vi "xijk_select_best_filter_remove_NaN.vi"(8 "error in":errorcluster, 10 "table_input_1D":string[](array[string]), 11 "table_input_2D":string[][](array[string])) -> (0 "error out":errorcluster, 2 "table_output_1D":string[](array[string]), 3 "table_output_2D":string[][](array[string]))   [LabVIEW 2009, in "xijk_select_best_filter.lvlib"]
uses:
  xijk_select_best_filter.lvlib
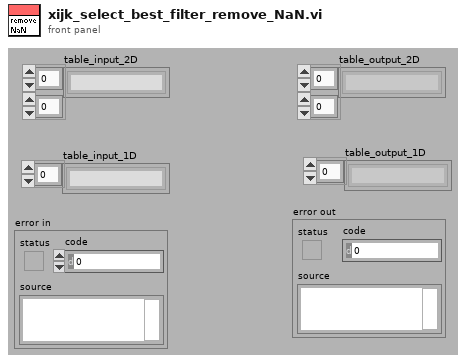
[diagram p1: front panel]
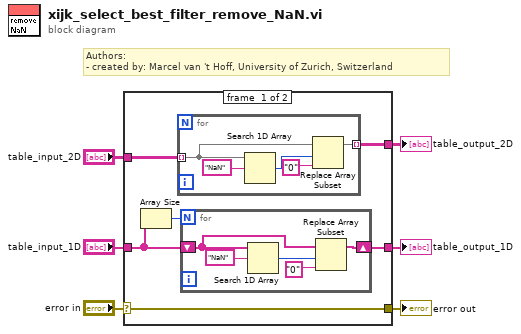
[diagram p0: block diagram]
diagram:
  # "Authors: \n- created by: Marcel van 't Hoff, University of Zurich, Switzerland"
  n1 = case shown="No Error" "error in" {
    selector: "error in" -> [w7 w23]
    tunnel: "table_input_2D" -> [w12 _]
    tunnel: [w11 _] -> w5
    tunnel: [w10 _] -> w4
    tunnel: "table_input_1D" -> [w9 _]
    tunnel: [w7 w23] -> w1
    frame #0 {
      n2 = Array Size(array=w9) -> (size(s)=w8:i32)
      n3 = for {
        tunnel: w12 -> [w21] mode=indexing
        tunnel: [w18] -> w11 mode=indexing
        n4 = Search 1D Array(1D array=w21, element="NaN" ("élément")) -> (index of element=w20:i32)  [unwired: 1 out]
        n5 = Replace Array Subset(array=w21, new element="0" ("nouvel élément/sous-tableau"), index=w20) -> (w18:string[])
      }
      n6 = for {
        N: w8 -> [_]
        shift-right: [w14] -> w10
        shift-left: w9 -> [w13]
        n7 = Search 1D Array(1D array=w13, element="NaN" ("élément")) -> (index of element=w16:i32)  [unwired: 1 out]
        n8 = Replace Array Subset(array=w13, new element="0" ("nouvel élément/sous-tableau"), index=w16) -> (w14:string[])
      }
    }
    frame #1 {
    }
  }
  "table_output_2D" <- w5
  "table_output_1D" <- w4
  "error out" <- w1
